vi "Read register value.vi"() -> ()   [LabVIEW 2011]
uses:
  <vilib>/registry/registry.llb/Registry RtKey.ctl
  <vilib>/registry/registry.llb/Read Registry Value Simple STR.vi
panel:
  out "String/Binary data":string
  out "Cluster":T1
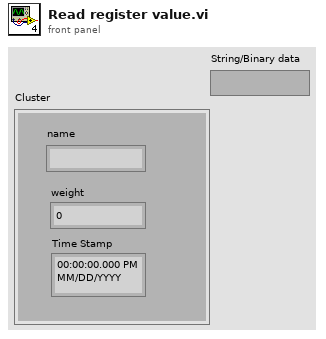
[diagram p1: front panel]
types:
  T1 = cluster{"name":string, "weight":i64, "Time Stamp":timestamp}
  T2 = typedef "Registry RtKey.ctl" = enum32{"HKEY_CLASSES_ROOT", "HKEY_CURRENT_USER", "HKEY_LOCAL_MACHINE", "HKEY_USERS", "HKEY_PERFORMANCE_DATA", "HKEY_CURRENT_CONFIG", "HKEY_DYN_DATA"}
  T3 = typedef "Registry refnum.ctl" = refnum<k1>
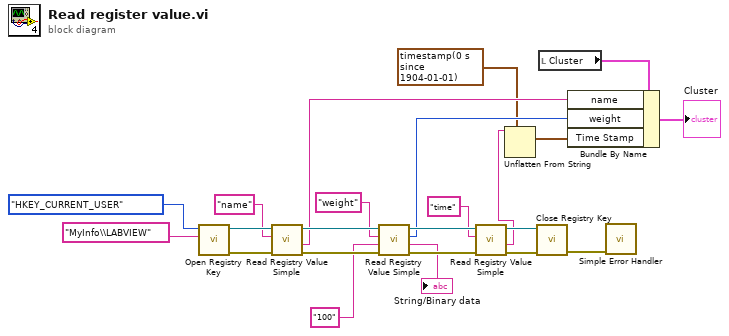
[diagram p0: block diagram]
diagram:
  n1 = call <vilib>:"Open Registry Key.vi"("subkey"="MyInfo\\LABVIEW", "root key (HKEY_LOCAL_MACHINE)"=Registry_RtKey."HKEY_CURRENT_USER") -> ("error out"=w22:errorcluster, "refnum out"=w23:T3)  [unwired: 8 in]
  n2 = call-poly <vilib>:"Read Registry Value Simple.vi"("error in (no error)"=w22, "value"="name", "refnum"=w23) -> ("error out"=w21:errorcluster, "String/Binary data"=w7:string, "refnum out"=w20:T3)  [unwired: 3 in, 1 out]
  n3 = call-poly <vilib>:"Read Registry Value Simple.vi"("error in (no error)"=w21, "default data"="100", "value"="weight", "refnum"=w20) -> ("error out"=w18:errorcluster, "String/Binary data"=→"String/Binary data":string, "simple data type"=w6:enum16{"String", "Binary", "DWORD"}, "refnum out"=w19:T3)  [unwired: 2 in]
  n4 = call-poly <vilib>:"Read Registry Value Simple.vi"("error in (no error)"=w18, "value"="time", "refnum"=w19) -> ("error out"=w17:errorcluster, "String/Binary data"=w3:string, "refnum out"=w16:T3)  [unwired: 3 in, 1 out]
  n5 = Unflatten From String(type=timestamp(0 s since 1904-01-01), binary string=w3) -> (value=w4:timestamp)  [unwired: 3 in, 2 out]
  n6 = call <vilib>:"Close Registry Key.vi"("error in (no error)"=w17, "refnum"=w16) -> ("error out"=w15:errorcluster)  [unwired: 5 in]
  n7 = local read "Cluster"() -> (w9:T1)
  n8 = Bundle By Name(cluster=w9, "name"=w7, "weight"=w6, "Time Stamp"=w4) -> (→"Cluster":T1)
  n9 = call <vilib>:"Simple Error Handler.vi"("error in (no error)"=w15) -> ()  [unwired: 4 in, 5 out]
